vi "Display.vi"(8 "error in":errorcluster, 11 "Gif - One Button in":refnum<class "Gif - One Button.lvclass">) -> (0 "error out":errorcluster, 3 "Gif - One Button out":refnum<class "Gif - One Button.lvclass">)   [LabVIEW 2021, in "Gif - One Button.lvclass"]
doc: "This is the override method required for each child of the pop up class. It is the pop up that will display to the user.\n\nTo extend this function, create a child class of the pop up class. Then create an override method for this VI. <b>Display.vi</b> is a protected function, therefore it cannot be called in a main application. This VI must be called by a caller function. See one of the standard pop-ups for a setup example.\n\n<b>Code Developed By:</b>\nDaniel Coons\nTechnology Service Corporation\n1983 S Liberty Drive\nBloomington, IN 47403\nPhone: 812 558-7100\ndaniel.coons@tsc.com\nwww.tsc.com/atcs"
uses:
  Gif - One Button.lvclass
  C:/Program Files/National Instruments/LabVIEW 2024/vi.lib/addons/_TSC/TSC Pop-Up/Popup/Popup.lvclass
  C:/Development/tsc-pop-up-gif/GIF Parent.lvclass
  <vilib>/addons/_TSC/TSC Pop-Up/Popup/Popup.lvclass/Popup.ctl
  GIF Parent.lvclass/GIF Parent.ctl
  <vilib>/addons/_TSC/TSC Pop-Up/Popup/Data Member Access/Read Theme.vi
  Read Delays.vi
  Read Gif Images.vi
  <vilib>/addons/_TSC/TSC Pop-Up/Theme/Theme.lvclass
  <vilib>/addons/_TSC/TSC Pop-Up/Popup/Popup.lvclass
  user32.dll
panel:
  in  "closer":bool
  out "header":bool
  out "Message":string
  out "2D Picture":picture
  in  "OK":bool
  # "This VI displays the popup"
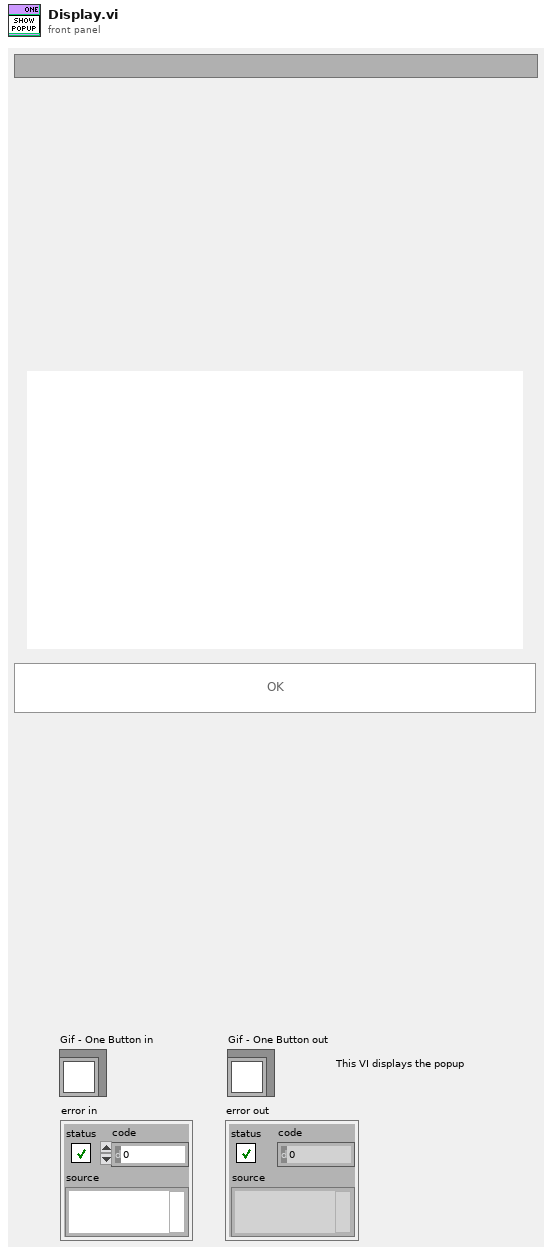
[diagram p1: front panel]
types:
  T1 = typedef "LVPoint32TypeDef.ctl" = cluster{"Horizontal":i32, "Vertical":i32}
  T2 = typedef "LVPositionTypeDef.ctl" = cluster{"Left":i32, "Top":i32}
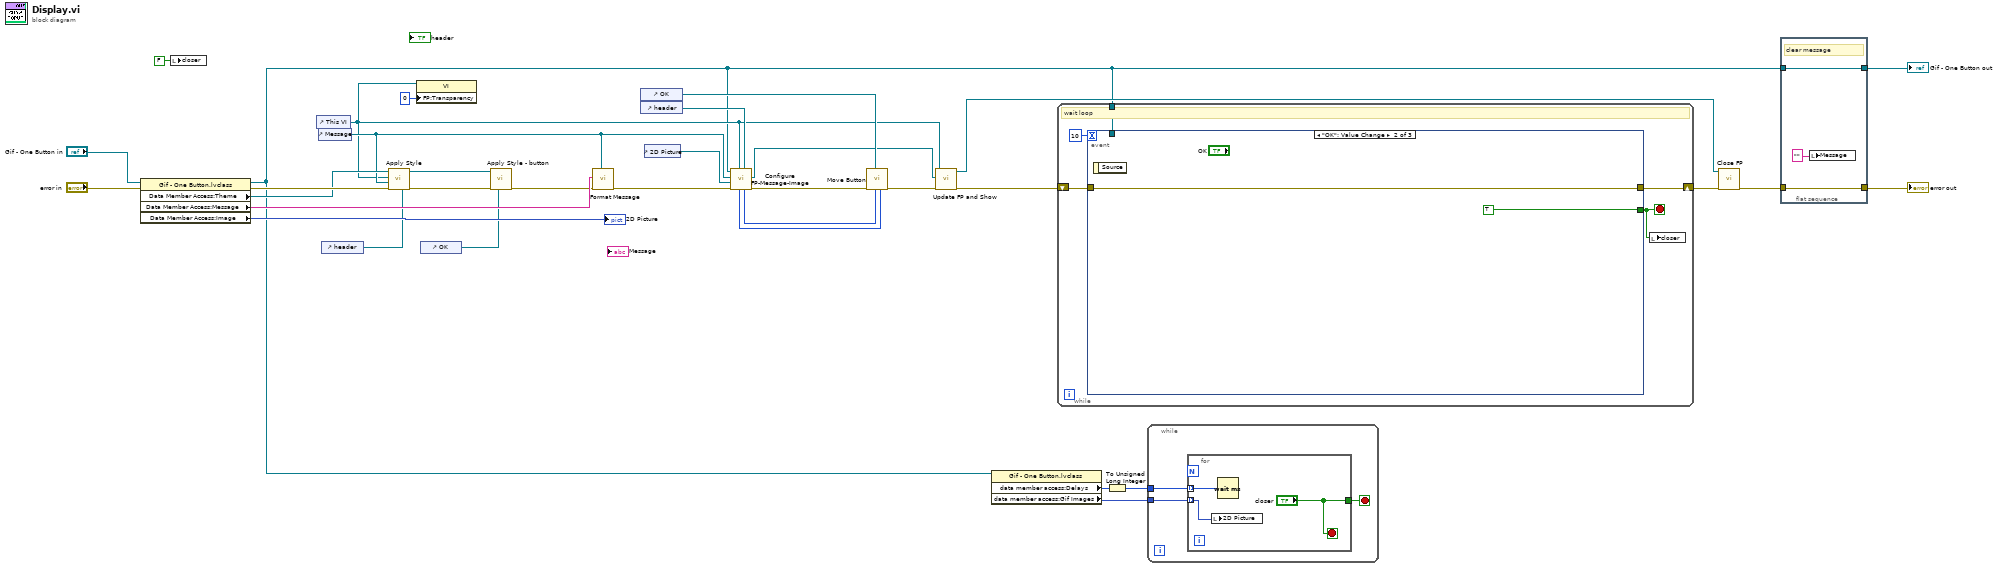
[diagram p0: block diagram]
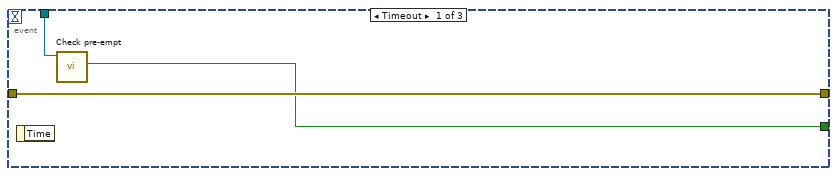
[diagram p2: hidden frame]
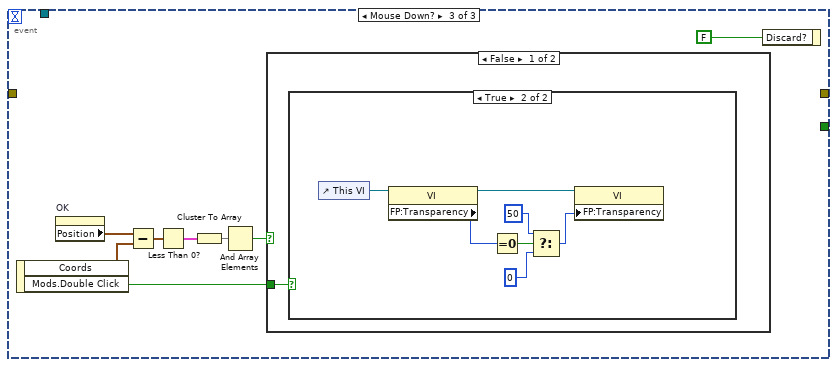
[diagram p3: hidden frame]
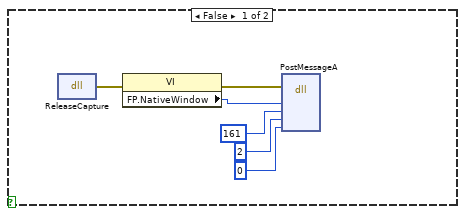
[diagram p4: hidden frame]
diagram:
  n1 = property class="Gif - One Button.lvclass"(reference="Gif - One Button in", error in="error in") -> (reference out=w1:refnum<class "Gif - One Button.lvclass">, error out=w34:errorcluster, "Data Member Access:Theme"=w29:refnum<class "Theme.lvclass">, "Data Member Access:Message"=w27:string, "Data Member Access:Image"=→"2D Picture":picture)
  n2 = local write "closer"(FALSE ("closer")) -> ()
  n3 = control-ref of="This VI"() -> (w11:refnum<vi>)
  n4 = control-ref of="Message"() -> (w23:refnum<vi>)
  n5 = control-ref of="header"() -> (w15:refnum<vi>)
  n6 = call <vilib>:"Apply Style.vi"("header ref"=w15, "error in (no error)"=w34, "message ref"=w23, "pop up ref"=w11, "Theme in"=w29) -> ("error out"=w17:errorcluster, "Theme out"=w26:refnum<class "Theme.lvclass">)  [unwired: 5 in]
  n7 = property class="VI"(reference=w11, "FP:Transparency"=u8 0 ("Front Panel Window:Transparency")) -> ()  [unwired: 1 in, 2 out]
  n8 = control-ref of="OK"() -> (w25:refnum<vi>)
  n9 = call <vilib>:"Apply Style - button.vi"("button ref"=w25, "error in (no error)"=w17, "Theme in"=w26) -> ("error out"=w16:errorcluster)  [unwired: 7 in, 1 out]
  n10 = call <vilib>:"Format Message.vi"("formatted string"=w23, "error in"=w16, "String Input"=w27) -> ("error out"=w13:errorcluster)  [unwired: 7 in, 1 out]
  n11 = control-ref of="OK"() -> (w24:refnum<vi>)
  n12 = control-ref of="header"() -> (w18:refnum<vi>)
  n13 = control-ref of="2D Picture"() -> (w22:refnum<vi>)
  n14 = call <vilib>:"Configure FP-Message-Image.vi"("header ref"=w18, "Pop Up ref"=w11, "error in (no error)"=w13, "Image ref"=w22, "Message ref"=w23, "Popup in"=w1) -> ("error out"=w14:errorcluster, "Panel Ref"=w19:refnum<vi>, "Panel Width"=w21:i32, "Panel Height"=w20:i32)  [unwired: 1 in, 1 out]
  n15 = call <vilib>:"Move Button.vi"("Panel Height"=w20, "Panel Width"=w21, "Button"=w24, "Error In"=w14) -> ("Error Out"=w33:errorcluster)  [unwired: 6 in, 1 out]
  n16 = call <vilib>:"Update FP and Show.vi"("error in (no error)"=w33, "Panel Ref"=w19, "VI in"=w11) -> ("error out"=w30:errorcluster, "VI out"=w12:refnum<vi>)  [unwired: 7 in]
  n17 = property class="Gif - One Button.lvclass"(reference=w1) -> ("data member access:Delays"=w5:i32[], "data member access:Gif Images"=w4:picture[])  [unwired: 1 in, 2 out]
  n18 = while {
    shift-right: [w39] -> w32
    shift-left: w30 -> [w38]
    tunnel: w1 -> [w36]
    stop <- w35 stop-if-true
    # "wait loop"
    n19 = event shown="[1] \"OK\": Value Change" {
      selector: _ -> [_ _ _]
      dyn-events: _ -> [_ _ _]
      timeout: 10 -> [_ _ _]
      tunnel: w38 -> [w42 w44 _]
      tunnel: [w42 w44 _] -> w39
      tunnel: [w40 TRUE _] -> w35
      tunnel: w36 -> [w41 _ _]
      event Timeout {
        n20 = event-data() -> ()  [unwired: 1 in, 1 out]
        n21 = call <vilib>:"Check pre-empt.vi"("_Popup in"=w41) -> ("Pre-empted?"=w40:bool)  [unwired: 8 in, 2 out]
      }
      event "OK": Value Change {
        n22 = event-data() -> ()  [unwired: 1 in, 1 out]
      }
      event Mouse Down? {
        n23 = event-data() -> ("Coords"=w45:T1, "Mods.Double Click"=w46:bool)  [unwired: 1 in]
        n24 = property on="OK" class="Bool"() -> ("Position"=w47:T2)  [unwired: 2 in, 2 out]
        n25 = Subtract(x=w47, y=w45) -> (x-y=w48:T2)
        n26 = Less Than 0?(x=w48) -> (x < 0?=w49:cluster{"Left":bool, "Top":bool})
        n27 = Cluster To Array(cluster=w49) -> (array=w50:bool[])
        n28 = And Array Elements(Boolean array=w50) -> (logical AND=w51:bool)
        n29 = case shown="False" w51 {
          tunnel: w46 -> [w53 _]
          frame False {
            n30 = case shown="True" w53 {
              frame False {
                n31 = dll-call lib="user32.dll" fn="ReleaseCapture"() -> (error out=w57:errorcluster)  [unwired: 4 in, 1 out]
                n32 = property class="VI"(error in=w57) -> (error out=w58:errorcluster, "FP.NativeWindow"=w59:u64)  [unwired: 1 in, 1 out]
                n33 = dll-call lib="user32.dll" fn="PostMessageA"(error in=w58, "hWnd"=w59, "Msg"=161, "wParam"=2, "lParam"=0) -> ()  [unwired: 7 in, 2 out]
              }
              frame True {
                n34 = control-ref of="This VI"() -> (w66:refnum<vi>)
                n35 = property class="VI"(reference=w66) -> (reference out=w64:refnum<vi>, "FP:Transparency"=w65:u8)  [unwired: 1 in, 1 out]
                n36 = Equal To 0?(x=w65) -> (x = 0?=w63:bool)
                n37 = Select(t=u8 50, s=w63, f=u8 0) -> (s? t:f=w62:u8)
                n38 = property class="VI"(reference=w64, "FP:Transparency"=w62) -> ()  [unwired: 1 in, 2 out]
              }
            }
          }
          frame True {
          }
        }
        n39 = event-data("Discard?"=FALSE) -> ()  [unwired: 1 in, 1 out]
      }
    }
    n40 = local write "closer"(w35) -> ()
  }
  n41 = To Unsigned Long Integer(number=w5) -> (unsigned 32bit integer=w2:u32[])
  n42 = while {
    tunnel: w2 -> [w68]
    tunnel: w4 -> [w67]
    stop <- w69 stop-if-true
    n43 = for {
      tunnel: ["closer"] -> w69
      tunnel: w68 -> [w71] mode=indexing
      tunnel: w67 -> [w70] mode=indexing
      stop <- "closer" stop-if-true
      n44 = local write "2D Picture"(w70) -> ()
      n45 = Wait (ms)(milliseconds to wait=w71) -> ()  [unwired: 1 out]
    }
  }
  n46 = call <vilib>:"Close FP.vi"("error in (no error)"=w32, "VI in"=w12) -> ("error out"=w31:errorcluster)  [unwired: 9 in]
  n47 = flat-sequence {
    tunnel: w31 -> [w75]
    tunnel: [w75] -> w6
    tunnel: w1 -> [w74]
    tunnel: [w74] -> w7
    frame #0 {
      # "clear message"
      n48 = local write "Message"("" ("Message")) -> ()
    }
  }
  "error out" <- w6
  "Gif - One Button out" <- w7
